vi "gyro -- async fitter.vi"(11 "fitter event pair":T9) -> ()   [LabVIEW 2021]
uses:
  lorentzian.ctl
  circle corners.ctl
  peak -- parameters -- complex fit.ctl
  wavepacket.ctl
  filter method control.ctl
  show-win- control.ctl
  server talk-to-back pair.ctl
  server talkback message type.ctl
  server talkto message type.ctl
  cursor winow.ctl
  plot refs -- filter related.ctl
  cursor window action.ctl
  publisher action.ctl
  arr action.ctl
  cursor action.ctl
  2Dwindow.ctl
  four-corner circle transformation.ctl
  filter - complex - four.vi
  linear interp iiii- complex - z-omega.vi
  peak -- PM find lorenzian - V3.vi
  Q -- check range -- i -- real.vi
  replace cursor action stack.vi
  Q -- range multiplier -- real -- V2.vi
  Q - not nan and gtr than zero - Real.vi
  Q - not nan -- real.vi
  array - smart min max.vi
  tale of three indices.vi
  filter -- window span logic.vi
  linear interp iiii- complex - z-omega - divide.vi
  linear interpolation iiii- complex.vi
  containing bix.vi
  <vilib>/Analysis/baseanly.llb/A x B.vi
  <vilib>/Analysis/baseanly.llb/Complex A x B.vi
  line -- complex.vi
  Q -- check range -- i -- integer.vi
  peak -- guess at omega -- dzdomega V2.vi
  command stack.vi
  tale of three indices -- check state.vi
  Q - not nan -- integer.vi
  peak -- z center from mult phase points.vi
  peak -- estimate for lorentzian.vi
  peak -- fake phase around center.vi
  peak -- get weights.vi
  peak -- four corner circle transformation logic.vi
  peak - fit phase around center - V2.vi
  array - generate range.vi
  circle center from three points.vi
  <vilib>/Utility/error.llb/Clear Errors.vi
  peak -- fit function -- minus arctan.vi
  <vilib>/Analysis/Matrix/Numeric/Conversions/Array To Matrix.vi
  <vilib>/Analysis/Matrix/Numeric/Conversions/Array To Matrix - RA2.vi
  <vilib>/Analysis/baseanly.llb/Inverse Matrix.vi
  <vilib>/Analysis/baseanly.llb/Real Inverse Matrix.vi
  <vilib>/gmath/NumericalOptimization/Nonlinear Curve Fit.vi
  <vilib>/gmath/NumericalOptimization/Nonlinear Curve Fit LM.vi
  KM_filter pipe - plot staff - more - V3.vi
panel:
  in  "Tab :  Fit controls":T1(tab)
  out "lorentzian":T2={"A (VHz)"=0.00528140496001674, "ω (Hz)"=0.00023844547824536982, "Γ (Hz)"=0.8041391285680035, "φ (rad)"=1.5732633738560469, "Q"=0.0002965226660092878, "Norm  Ampl"=nan, "z∞ (V)"=0.027690666556369502-1.7738793870681028e-05i, "4corners"={"z (-pi/2)"=0.03424221869371515+0.006566219331209036i, "z(inf)"=0.027690666556369502-1.7738793870681028e-05i, "z (pi/2)"=0.03427462468144921-0.0065692909312163265i, "z center"=0.03425842168758218-1.535800003645652e-06i, "z(0)"=0.040826176818794864+1.4667193863389723e-05i, "radius"=0.006567775117997019}} {"z∞ (V)" format="%#_4p"; "Q" format="%#_4p"; "φ (rad)" format="%#_3p"; "Γ (Hz)" format="%#_5p"; "ω (Hz)" format="%#_9p"; "A (VHz)" format="%#_3p"}
  in  "Plot: fragment - filter":cluster{dbl[], dbl[]}[](graph)=[{array[1567 elements], array[1567 elements]}, {array[1567 elements], array[1567 elements]}, {array[1567 elements], array[1567 elements]}, {array[1567 elements], array[1567 elements]}]
  out "Plot: phase around center":cluster{dbl[], dbl[]}[](graph)
  out "Plot: fragment":cluster{dbl[], dbl[]}[](graph)
  out "Plot: complex plane":cluster{dbl[], dbl[]}[](graph)=[{array[1567 elements], array[1567 elements]}, {[0.0408261968055792, 0.04077440793707446, 0.04061985807295371, 0.04036498455689775, 0.040013806896508845, 0.039571863373274695, 0.03904612370056097, 0.038444879107068015, 0.03777761157920133, 0.03705484432448167, 0.03628797581427619, 0.035489100023095875, 0.03467081569939291, 0.03384602767577145, 0.03302774335206849, 0.03222886756088818, 0.0314619990506827, 0.030739231795963037, 0.03007196426809635, 0.029470719674603397, 0.02894498000188967, 0.02850303647865552, 0.02815185881826662, 0.027896985302210662, 0.02774243543808991, 0.027690646569585163, 0.02774243543808991, 0.027896985302210662, 0.02815185881826662, 0.02850303647865552, 0.02894498000188967, 0.029470719674603397, 0.030071964268096354, 0.03073923179596304, 0.031461999050682705, 0.03222886756088818, 0.03302774335206849, 0.03384602767577145, 0.03467081569939291, 0.03548910002309588, 0.03628797581427619, 0.03705484432448167, 0.03777761157920133, 0.038444879107068015, 0.03904612370056097, 0.0395718633732747, 0.040013806896508845, 0.04036498455689775, 0.04061985807295371, 0.04077440793707446], [-1.535800003645652e-06, 0.0008216246928581006, 0.001631803453015174, 0.002416223477442565, 0.0031625139937652446, 0.0038589055547284595, 0.004494415649411666, 0.00505902190398638, 0.00554382014053853, 0.005941164801273261, 0.006244789523528591, 0.006449905964057936, 0.006553279314063525, 0.006553279314063525, 0.006449905964057935, 0.00624478952352859, 0.005941164801273261, 0.005543820140538529, 0.005059021903986379, 0.004494415649411665, 0.00385890555472846, 0.003162513993765244, 0.0024162234774425632, 0.001631803453015174, 0.0008216246928580996, -1.5358000036477643e-06, -0.0008246962928653923, -0.0016348750530224665, -0.0024192950774498587, -0.003165585593772537, -0.003861977154735753, -0.0044974872494189565, -0.005062093503993671, -0.005546891740545822, -0.005944236401280553, -0.006247861123535881, -0.006452977564065226, -0.006556350914070815, -0.006556350914070815, -0.0064529775640652254, -0.0062478611235358816, -0.005944236401280552, -0.00554689174054582, -0.005062093503993669, -0.004497487249418954, -0.0038619771547357476, -0.0031655855937725366, -0.0024192950774498557, -0.0016348750530224632, -0.0008246962928653888]}, {[0.027690666556369502, 0.02834744206949077, 0.029004217582612037, 0.029660993095733307, 0.030317768608854573, 0.030974544121975842, 0.03163131963509711, 0.03228809514821838, 0.032944870661339644, 0.03360164617446092, 0.03425842168758218, 0.03491519720070345, 0.035571972713824715, 0.03622874822694599, 0.036885523740067254, 0.03754229925318853, 0.03819907476630979, 0.03885585027943106, 0.039512625792552325, 0.0401694013056736], [-1.7738793870681028e-05, -1.611849448397749e-05, -1.4498195097273952e-05, -1.2877895710570416e-05, -1.1257596323866877e-05, -9.63729693716334e-06, -8.016997550459804e-06, -6.396698163756265e-06, -4.7763987770527285e-06, -3.1560993903491917e-06, -1.5358000036456533e-06, 8.449938305788346e-08, 1.7047987697614202e-06, 3.325098156464957e-06, 4.945397543168497e-06, 6.565696929872034e-06, 8.18599631657557e-06, 9.806295703279107e-06, 1.1426595089982644e-05, 1.304689447668618e-05]}, {[0.03424221869371515, 0.034243838993101856, 0.03424545929248856, 0.034247079591875264, 0.03424869989126197, 0.034250320190648664, 0.03425194049003537, 0.03425356078942207, 0.034255181088808775, 0.03425680138819548, 0.03425842168758218, 0.03426004198696889, 0.03426166228635559, 0.034263282585742294, 0.034264902885129, 0.0342665231845157, 0.0342681434839024, 0.0342697637832891, 0.034271384082675806, 0.03427300438206251], [0.006566219331209036, 0.005909443818087768, 0.005252668304966499, 0.004595892791845232, 0.003939117278723963, 0.003282341765602695, 0.0026255662524814274, 0.001968790739360159, 0.001312015226238891, 0.0006552397131176233, -1.5358000036453517e-06, -0.0006583113131249131, -0.0013150868262461809, -0.0019718623393674486, -0.002628637852488718, -0.003285413365609986, -0.003942188878731254, -0.0045989643918525214, -0.005255739904973789, -0.005912515418095059]}, {[0.161429891576008, 0.16228628660951472, 0.1630599306451906, 0.16375034018069645, 0.16435708373254648, 0.16487978210577106, 0.16531810863090154, 0.16567178936812785, 0.16594060327850202, 0.16612438236208033, 0.16622301176291782, 0.1662364298408495, 0.16616462821001343, 0.16600765174409163, 0.1657655985482655, 0.1654386198979033, 0.16502692014401782, 0.16453075658555388, 0.16395043930858472, 0.16328633099251824], [-0.035709224864324776, -0.0324095456256249, -0.02908948983727056, -0.02575113242605699, -0.022396559756697982, -0.019027868327915826, -0.015647163462197872, -0.012256557990038502, -0.008858170929488846, -0.005454126161839468, -0.0020465511042637103, 0.0013624246197488027, 0.004770670511337509, 0.008176056527763353, 0.011576454413616181, 0.01496973903090505, 0.01835378968720035, 0.021726491460997498, 0.02508573652347404, 0.028429425455814096]}, {[0.17590062231507544, 0.17685122080226792, 0.17770996568186812, 0.17847632026627963, 0.17914980560883315, 0.17973000080311247, 0.1802165432460073, 0.18060912886432848, 0.1809075123048438, 0.18111150708761575, 0.18122098572254536, 0.1812358797890495, 0.18115617997882147, 0.18098193610164828, 0.1807132570542813, 0.18035031075237923, 0.17989332402556635, 0.1793425824756714, 0.1786984302982356, 0.1779612700674018], [-0.039658649110643325, -0.03599600515568646, -0.03231074323061314, -0.02860516650416608, -0.024881590841177584, -0.021142343355229392, -0.017389760954282463, -0.01362618888018556, -0.00985397924297544, -0.006075489550884631, -0.00229308123697554, 0.0014908818166783503, 0.005274034756341815, 0.009054013234574502, 0.01282845488787114, 0.016595000813061783, 0.02035129704154957, 0.024094996010464404, 0.027823758029813368, 0.031535252744710834]}, {array[1567 elements], array[1567 elements]}]
  in  "scale gauge: Plot: complex plane":dbl(slide)=0.00275 min=0.0 max=0.3 step=1e-06 scale=1e-06..5000000000.0 scale format="%#_3p"
  out "Plot: phase":cluster{"omega out":dbl[], dbl[]}(graph)
  out "Plot: win omega":T4(graph)
  out "Plot: dz/domega":cluster{"omega out":dbl[], dbl[]}(graph)
  in  "Plot: complex plane - filter":cluster{dbl[], dbl[]}[](graph)=[{array[1567 elements], array[1567 elements]}, {array[1567 elements], array[1567 elements]}, {[0.041161284502408316, 0.04114804194794312, 0.04110836654686009, 0.041042414879841324, 0.04095044722798609, 0.040832826545600234, 0.04069001702778137, 0.04052258227845285, 0.040331183086076625, 0.04011657481582302, 0.03987960442848954, 0.03962120713793352, 0.039342402720210286, 0.039044291488982974, 0.038728049953087165, 0.038394926173388036, 0.03804623483725427, 0.037683352070087675, 0.03730771000438489, 0.0369207911277647, 0.03652412243226672, 0.03611926938801138, 0.0357078297650046, 0.0352914273274695, 0.03487170542559085, 0.034450320509962676, 0.0340289355943345, 0.03360921369245585, 0.03319281125492075, 0.03278137163191397, 0.03237651858765863, 0.03197984989216064, 0.03159293101554046, 0.031217288949837673, 0.030854406182671077, 0.030505714846537316, 0.030172591066838183, 0.029856349530942378, 0.029558238299715062, 0.02927943388199183, 0.02902103659143581, 0.02878406620410233, 0.028569457933848727, 0.0283780587414725, 0.028210623992143982, 0.028067814474325114, 0.027950193791939262, 0.027858226140084028, 0.02779227447306526, 0.027752599071982225, 0.02773935651751704, 0.027752599071982225, 0.02779227447306526, 0.027858226140084028, 0.027950193791939262, 0.028067814474325114, 0.028210623992143982, 0.0283780587414725, 0.028569457933848727, 0.028784066204102333, 0.02902103659143581, 0.029279433881991834, 0.029558238299715066, 0.029856349530942378, 0.030172591066838183, 0.030505714846537316, 0.03085440618267108, 0.031217288949837677, 0.03159293101554046, 0.03197984989216065, 0.03237651858765862, 0.03278137163191397, 0.03319281125492075, 0.033609213692455855, 0.0340289355943345, 0.034450320509962676, 0.03487170542559086, 0.0352914273274695, 0.035707829765004605, 0.03611926938801138, 0.03652412243226672, 0.03692079112776471, 0.03730771000438489, 0.03768335207008768, 0.03804623483725427, 0.03839492617338804, 0.03872804995308717, 0.039044291488982974, 0.03934240272021029, 0.03962120713793352, 0.03987960442848955, 0.04011657481582302, 0.040331183086076625, 0.04052258227845285, 0.04069001702778137, 0.04083282654560024, 0.04095044722798609, 0.041042414879841324, 0.04110836654686009, 0.04114804194794312], [0.0, 0.0004213849156281766, 0.0008411068175068247, 0.0012575092550419264, 0.0016689488780487088, 0.002073801922304048, 0.0024704706178020307, 0.002857389494422215, 0.0032330315601250014, 0.0035959143272915966, 0.003944605663425361, 0.004277729443124494, 0.004593970979020299, 0.004892082210247612, 0.005170886627970845, 0.005429283918526867, 0.005666254305860345, 0.005880862576113948, 0.006072261768490176, 0.006239696517818694, 0.006382506035637562, 0.0065001267180234135, 0.006592094369878648, 0.006658046036897418, 0.00669772143798045, 0.006710963992445636, 0.00669772143798045, 0.006658046036897418, 0.006592094369878648, 0.0065001267180234135, 0.006382506035637562, 0.006239696517818694, 0.006072261768490176, 0.005880862576113947, 0.005666254305860344, 0.005429283918526867, 0.005170886627970844, 0.004892082210247611, 0.004593970979020297, 0.004277729443124492, 0.003944605663425362, 0.0035959143272915966, 0.0032330315601250006, 0.002857389494422214, 0.002470470617802029, 0.0020738019223040458, 0.0016689488780487088, 0.001257509255041926, 0.0008411068175068236, 0.000421384915628175, -2.1584377821951928e-18, -0.0004213849156281764, -0.000841106817506825, -0.0012575092550419272, -0.00166894887804871, -0.00207380192230405, -0.002470470617802033, -0.0028573894944222147, -0.003233031560125002, -0.003595914327291598, -0.003944605663425363, -0.0042777294431244955, -0.004593970979020299, -0.004892082210247612, -0.005170886627970845, -0.005429283918526866, -0.0056662543058603465, -0.005880862576113948, -0.0060722617684901775, -0.006239696517818694, -0.006382506035637562, -0.006500126718023414, -0.006592094369878648, -0.006658046036897419, -0.006697721437980451, -0.006710963992445636, -0.00669772143798045, -0.006658046036897418, -0.006592094369878647, -0.0065001267180234135, -0.006382506035637563, -0.006239696517818693, -0.006072261768490176, -0.005880862576113946, -0.005666254305860345, -0.005429283918526863, -0.005170886627970843, -0.004892082210247612, -0.004593970979020296, -0.004277729443124492, -0.0039446056634253575, -0.003595914327291595, -0.0032330315601250014, -0.0028573894944222116, -0.00247047061780203, -0.0020738019223040436, -0.0016689488780487068, -0.0012575092550419268, -0.0008411068175068216, -0.00042138491562817583]}, {[-0.0011564988801927543, 0.004572526561840443, -0.002112059205125437], [0.00335441079091194, -0.0001946319203892838, 0.002611932143364084]}, {[-0.0013298665711747892, -0.00137040717662973, -0.0014109477820846707, -0.0014514883875396116, -0.0014920289929945525, -0.0015325695984494932, -0.001573110203904434, -0.001613650809359375, -0.0016541914148143159, -0.0016947320202692566, -0.0017352726257241974, -0.0017758132311791381, -0.001816353836634079, -0.00185689444208902, -0.0018974350475439608, -0.0019379756529989017, -0.001978516258453842, -0.002019056863908783, -0.002059597469363724, -0.002100138074818665], [0.002923118173286433, 0.002884411809776051, 0.002845705446265669, 0.0028069990827552867, 0.002768292719244905, 0.0027295863557345226, 0.0026908799922241403, 0.0026521736287137584, 0.002613467265203376, 0.0025747609016929943, 0.002536054538182612, 0.0024973481746722297, 0.002458641811161848, 0.0024199354476514656, 0.0023812290841410838, 0.0023425227206307015, 0.0023038163571203196, 0.0022651099936099373, 0.002226403630099555, 0.002187697266589173]}, {[0.004572526561840443, 0.004665772051033478, 0.0047590175402265145, 0.00485226302941955, 0.004945508518612586, 0.005038754007805622, 0.005131999496998658, 0.005225244986191694, 0.00531849047538473, 0.005411735964577766, 0.005504981453770801, 0.005598226942963838, 0.005691472432156874, 0.0057847179213499095, 0.005877963410542945, 0.0059712088997359814, 0.006064454388929017, 0.006157699878122053, 0.006250945367315089, 0.006344190856508124], [-0.0001946319203892838, -0.0001946319203892838, -0.0001946319203892838, -0.0001946319203892838, -0.0001946319203892838, -0.0001946319203892838, -0.0001946319203892838, -0.0001946319203892838, -0.0001946319203892838, -0.0001946319203892838, -0.0001946319203892838, -0.0001946319203892838, -0.0001946319203892838, -0.0001946319203892838, -0.0001946319203892838, -0.0001946319203892838, -0.0001946319203892838, -0.0001946319203892838, -0.0001946319203892838, -0.0001946319203892838]}]
  in  "parameters: complex fit":T5={"main VI path"=path "", "scale factor"=3.0, "# of grid points"=200, "parameters: wavepacket"={"R"=0.5, "wave number"=22.0, "delta k"=7.0, "radii vector"=[], "radial section"=[], "wave vector"=22.0, "wavepacket is"=TRUE}, "span"=0.27789, "interference ?"=enum."cp z center", "filter method"=enum."three"} {"span" min=0.0 max=0.5 step=1e-05 scale=0.0001..0.5 scale format="%#_5f"; "parameters: wavepacket"."delta k" format="%#_3f"; "parameters: wavepacket"."wave number" format="%#_3f"; "parameters: wavepacket"."R" format="%#_3f"}
  in  "win":T8={"cen (Hz)"=45005.0594236074, "win (Hz)"=127.23590686512762, "left (Hz)"=44941.44147017484, "right (Hz)"=45068.67737703997} {"right (Hz)" format="%#_3p"}
  out "circle frequency (Hz)":dbl=0.00023844547824536982 format="%#11_11f"
  out "circle gamma (Hz)":dbl=0.8041391285680035 format="%#11_11f"
  out "circle phase (rad)":dbl=1.5732633738560469 format="%#11_11f"
  out "circle Q":dbl=0.0002965226660092878 format="%#11_11f"
  in  "use fast fit!":bool
  in  "plot staff!":enum16{"plot", "do not plot", "a"}(ring)
  in  "cursor window":T10={"left"=0.0, "right "=0.0, "center"=0.0, "window"=0.0, "cursors"=[4, 5, 6], "relative"=0, "absolute"=0, "fixed vertical offset"=0.0, "vertical offset"=0.0, "skew"=0.0, "default window frac"=0.1, "kind"=enum."symmetric", "skew.left"=0.5, "skew.right"=0.5, "Plot ref"=refnum, "wing order"=enum."forw"}
  in  "tab":enum32{"complex plane"}(tab)
  out "# of points":dbl=953.475933538175
  out "center (kHz)":dbl=3399.029286744401
  out "win width (kHz)":dbl=76.27809365793496
  in  "ignore win":T8 {"right (Hz)" format="%#_3p"}
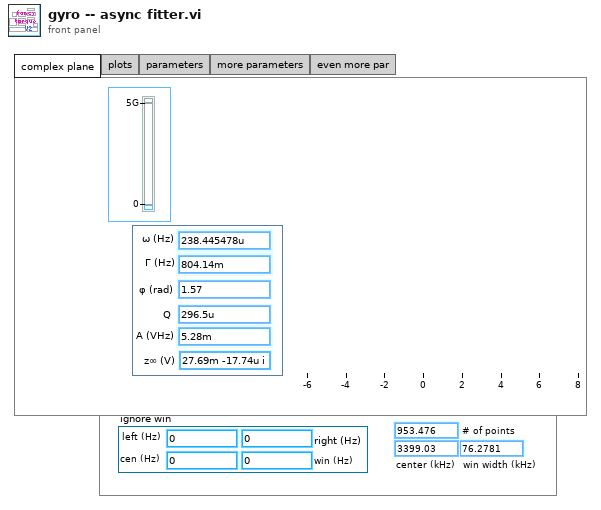
[diagram p1: front panel]
types:
  T1 = enum32{"complex plane", "plots", "parameters", "more parameters", "even more par"}
  T2 = typedef "lorentzian.ctl" = cluster{"A (VHz)":dbl, "ω (Hz)":dbl, "Γ (Hz)":dbl, "φ (rad)":dbl, "Q":dbl, "Norm  Ampl":dbl, "z∞ (V)":cdb, "4corners":T3}
  T3 = typedef "circle corners.ctl" = cluster{"z (-pi/2)":cdb, "z(inf)":cdb, "z (pi/2)":cdb, "z center":cdb, "z(0)":cdb, "radius":dbl}
  T4 = cluster{"omega out":dbl[], "win omega out":dbl[]}
  T5 = typedef "peak -- parameters -- complex fit.ctl" = cluster{"main VI path":path, "scale factor":dbl, "# of grid points":i32, "parameters: wavepacket":T6, "span":dbl, "interference ?":enum16{"cp z center", "pm zcenter", "fancy"}, "filter method":T7}
  T6 = typedef "wavepacket.ctl" = cluster{"R":dbl, "wave number":dbl, "delta k":dbl, "radii vector":dbl[], "radial section":cdb[], "wave vector":dbl, "wavepacket is":bool}
  T7 = typedef "filter method control.ctl" = enum16{"four", "five", "one", "two", "three", "zero", "minus one", "minus two"}
  T8 = typedef "show-win- control.ctl" = cluster{"cen (Hz)":dbl, "win (Hz)":dbl, "left (Hz)":dbl, "right (Hz)":dbl}
  T9 = typedef "server talk-to-back pair.ctl" = cluster{"talkback event":refnum<user-event>, "talkto event":refnum<user-event>}
  T10 = typedef "cursor winow.ctl" = cluster{"left":dbl, "right ":dbl, "center":dbl, "window":dbl, "cursors":i32[], "relative":i32, "absolute":i32, "fixed vertical offset":dbl, "vertical offset":dbl, "skew":dbl, "default window frac":dbl, "kind":enum16{"symmetric", "skewed", "fancy"}, "skew.left":dbl, "skew.right":dbl, "Plot ref":refnum<vi>, "wing order":enum16{"forw", "back"}}
  T11 = typedef "cursor window action.ctl" = enum16{"balance", "h. offset change", "cursor moves", "change center", "change window", "init", "check", "reset", "set y to middle", "idle", "-write all Y", "-write left.X", "-write center.X", "-write right.X", "-write all X", "-change center", "-change window", "-change skew", "-read cursor 2", "-read cursor 1", "-read cursor 0", "-read all cursors", "-reset", "-read plot scale", "-set y to middle", "-Q: center.Y is visible", "-Q: window is visible", "-parse center.Y", "-right left from center", "-left move", "-right move", "-set center.Y", "-empty", "-set cursors to default", "-check", "-write center.Y", "-copy cursor 1", "-copy cursor 0", "-copy cursor 2", "move right", "move left", "shrink", "broaden", "skew up", "skew down", "-write plot scale", "zoom X", "change cen&win", "zoom to all data", "color--red", "color--green", "color--yellow", "read", "zoom out", "zoom in", "slide right", "slide left", "set range aspect ratio to 1", "move to window range", "--move to window range"}
  T12 = enum16{"stop", "start", "update pars", "update request", "new", "launch", "exit", "get", "reset", "pause", "unpause"}
  T13 = typedef "plot refs -- filter related.ctl" = cluster{"Plot: complex plane - filter":refnum<vi>, "Plot: dz/domega":refnum<vi>, "Plot: fragment filter":refnum<vi>, "Plot: win omega":refnum<vi>, "Plot: phase":refnum<vi>, "Plot: phase around center":refnum<vi>, "Plot: complex plane":refnum<vi>, "Plot: fragment":refnum<vi>}
  T14 = typedef "arr action.ctl" = enum16{"select", "remove", "init", "check"}
  T15 = typedef "publisher action.ctl" = enum16{"set", "get", "init", "check"}
  T16 = typedef "server talkback message type.ctl" = cluster{"message":enum16{"new", "void"}}
  T17 = typedef "four-corner circle transformation.ctl" = enum16{"z(c) z(inf)", "z(c) z(zero)", "fix phase", "calculate lorentzian", "z(0) z(+-pi/2)", "shift to zcenter", "to  canonical", "get canonical phase", "get4corners", "update lorentzian -- from z0", "fake gamma normal", "fake gamma heat", "calculate complex slope", "get f0 given f and phi"}
  T18 = typedef "2Dwindow.ctl" = cluster{"window y":dbl, "center x":dbl, "center y":dbl, "window x":dbl}
  T19 = typedef "cursor action.ctl" = enum16{"range", "read", "write", "check", "zoom out", "smart zoom out", "zoom to aspect ratio 1", "zoom to win", "zoom out 20%", "zoom in 20%", "-empty", "smart zoom out&aspect", "move range left 20%", "move range right 20%", "move range up 20%", "move range down 20%", "zoom to X win", "zoom to Y win", "zoom out X", "zoom out Y", "zoom in X", "zoom in Y", "check plot scale", "set plot color", "set Xlabel", "set Ylabel", "set cursor color", "setlength", "empty", "hide plot", "unhide plot", "checklngth", "extend +1 if short", "extend +n if short"}
  T20 = typedef "eventvkey.ctl" = enum16{"ASCII", "Enter", "Return", "Shift", "Ctrl", "Alt", "Cmd", "Opt", "Caps", "NumLock", "Clear", "Break", "Up", "Down", "Left", "Right", "Insert", "Delete", "Home", "End", "PageUp", "PageDown", "Escape", "Help", "Pause", "ScrollLock", "F1", "F2", "F3", "F4", "F5", "F6", "F7", "F8", "F9", "F10", "F11", "F12", "F13", "F14", "F15", "F16", "F17", "F18", "F19", "F20", "F21", "F22", "F23", "F24", "Play", "VolumeUp", "VolumeDown", "Mute", "Two Byte Char"}
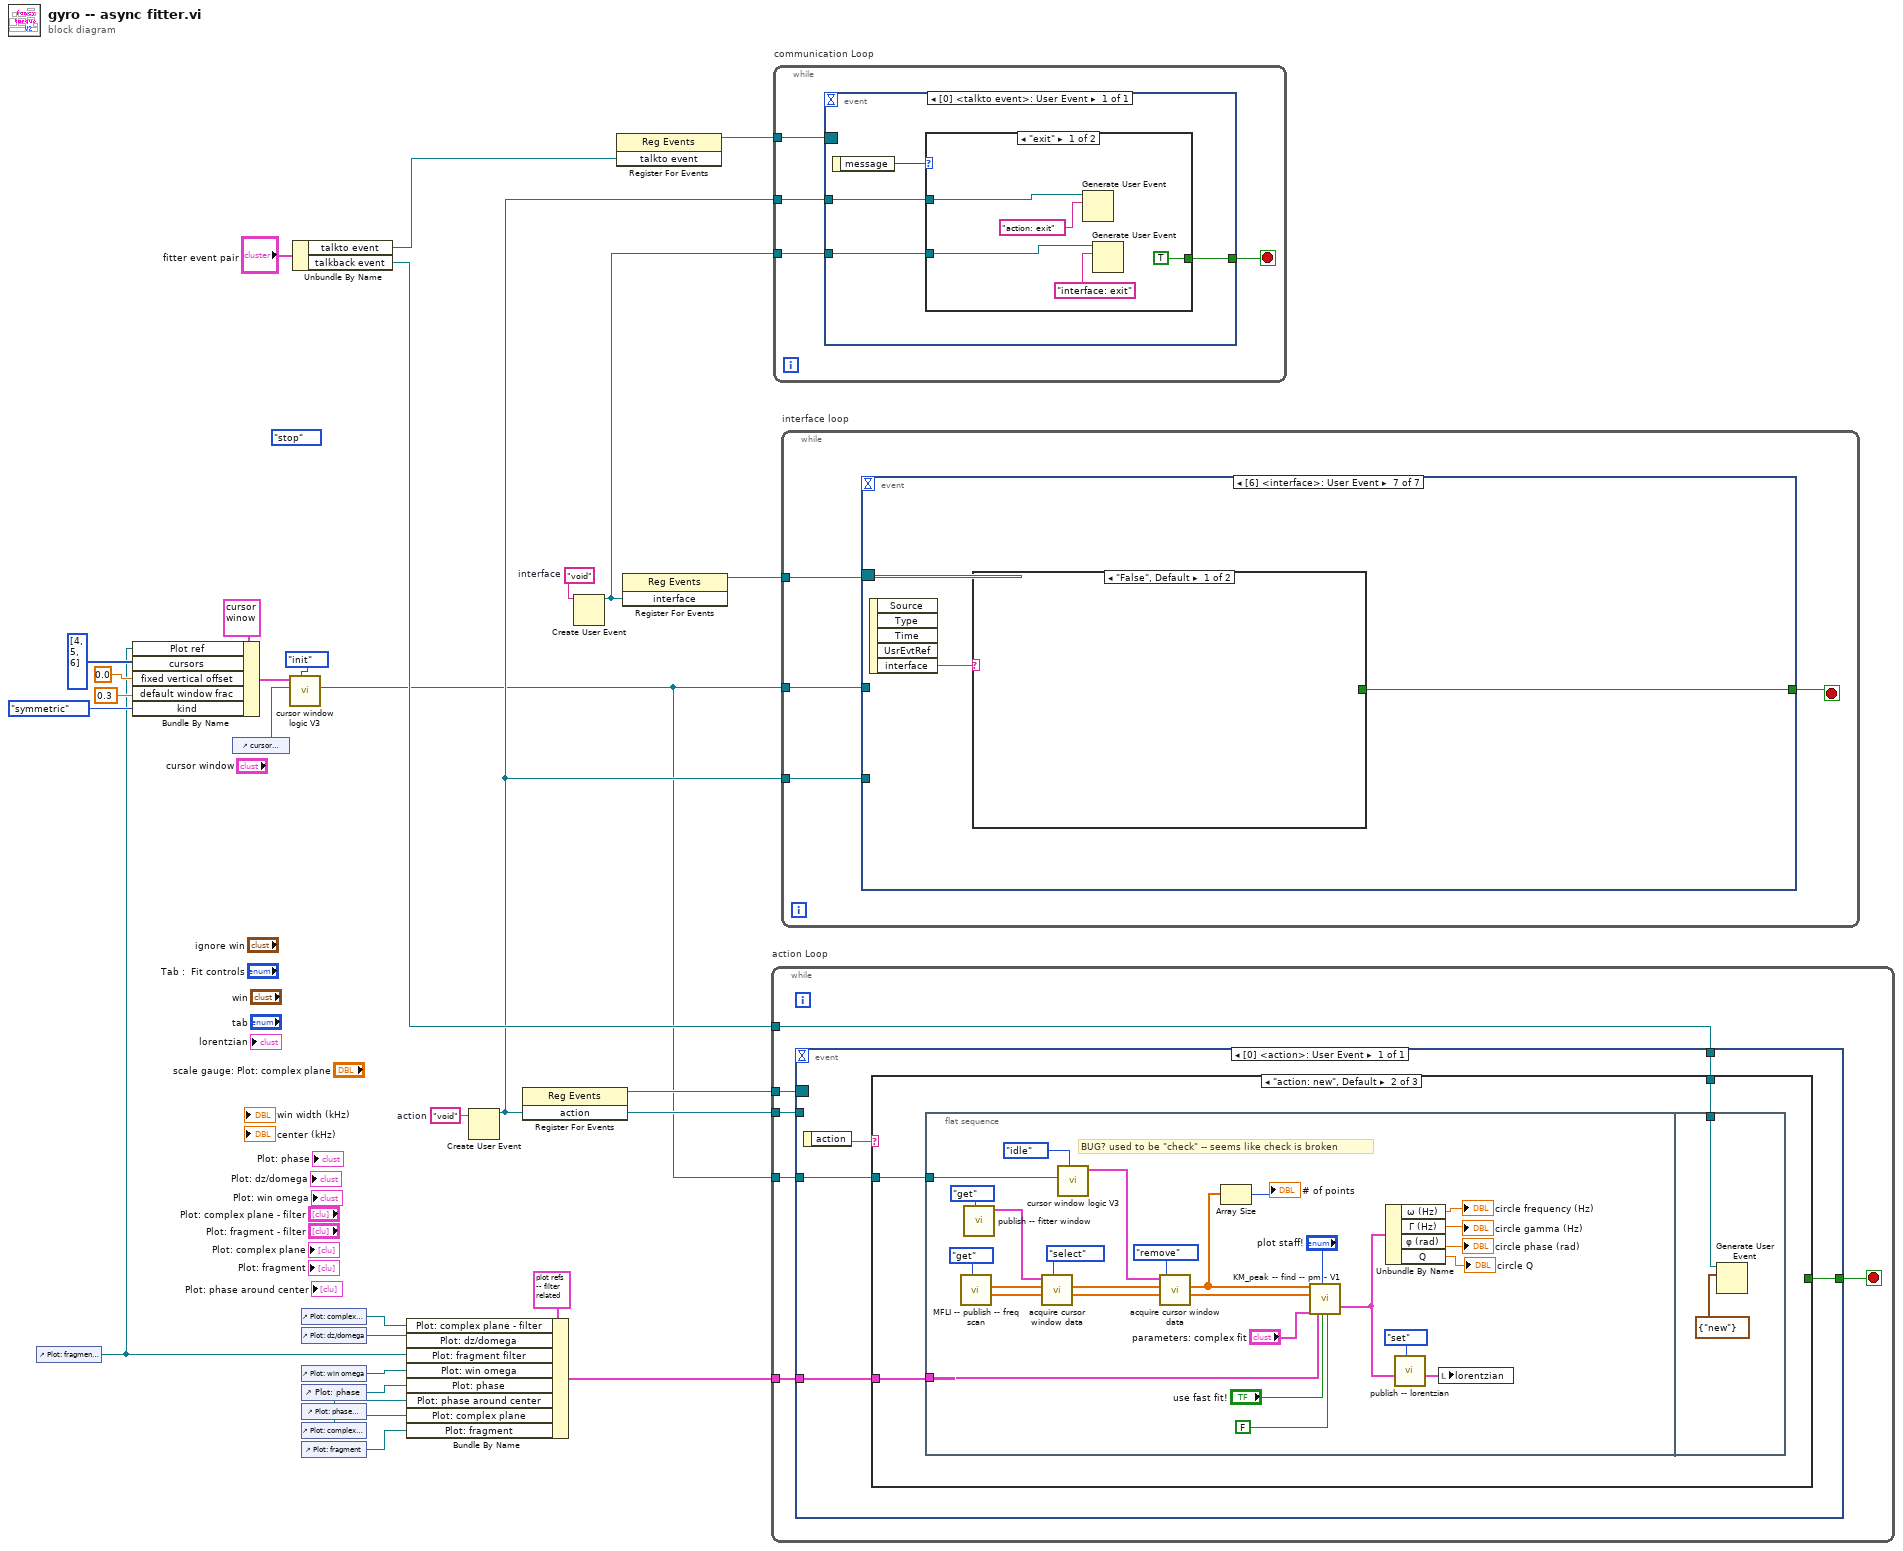
[diagram p0: block diagram]
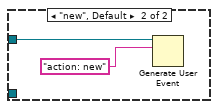
[diagram p2: hidden frame]
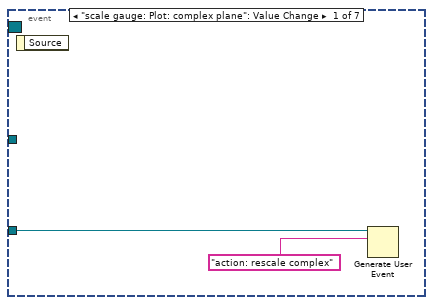
[diagram p3: hidden frame]
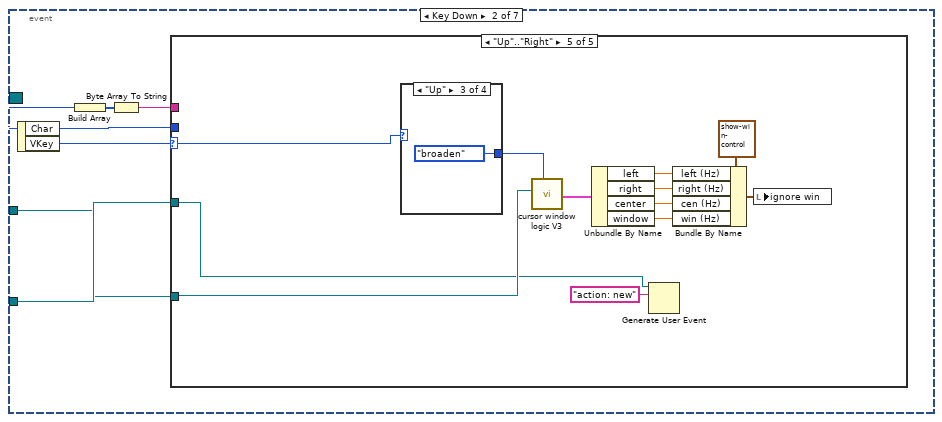
[diagram p4: hidden frame]
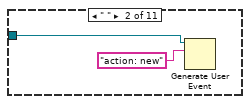
[diagram p6: hidden frame]
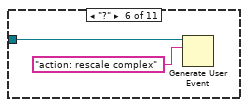
[diagram p10: hidden frame]
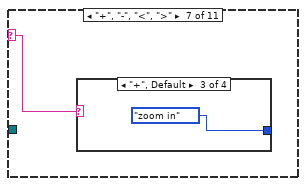
[diagram p11: hidden frame]
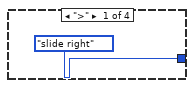
[diagram p12: hidden frame]
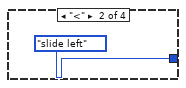
[diagram p13: hidden frame]
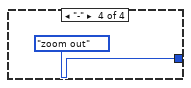
[diagram p14: hidden frame]
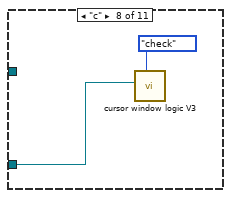
[diagram p15: hidden frame]
diagram:
  (unwired) T12."stop" ("message")
  w26 = "void"  # interface
  w28 = "void"  # action
  n1 = control-ref of="Plot: fragment - filter"() -> (w2:refnum<vi>)
  n2 = Bundle By Name(cluster=T10 {"left"=0.0, "right "=0.0, "center"=0.0, "window"=0.0, "cursors"=[], "relative"=0, "absolute"=0, "fixed vertical offset"=0.0, "vertical offset"=0.0, "skew"=0.0, "default window frac"=0.0, "kind"=enum."symmetric", "skew.left"=0.0, "skew.right"=0.0, "Plot ref"=refnum, "wing order"=enum."forw"} ("cursor bracket: All, data window"), "Plot ref"=w2, "cursors"=i32[] [4, 5, 6], "fixed vertical offset"=0.0, "default window frac"=0.3 ("fixed vertical offset"), "kind"=enum16{"symmetric", "skewed", "fancy"}."symmetric") -> (w6:T10)
  n3 = control-ref of="cursor window"() -> (w3:refnum<vi>)
  n4 = call "cursor window logic V3.vi"("cursor window action"=cursor_window_action."init", "cursor window in"=w3, "cursor window init"=w6) -> ("cursor window out"=w1:refnum<vi>)  [unwired: 7 in, 1 out]
  n5 = Unbundle By Name("fitter event pair") -> ("talkto event"=w14:refnum<user-event>, "talkback event"=w13:refnum<user-event>)
  n6 = control-ref of="Plot: complex plane - filter"() -> (w24:refnum<vi>)
  n7 = control-ref of="Plot: dz/domega"() -> (w23:refnum<vi>)
  n8 = control-ref of="Plot: win omega"() -> (w22:refnum<vi>)
  n9 = control-ref of="Plot: phase"() -> (w21:refnum<vi>)
  n10 = control-ref of="Plot: phase around center"() -> (w19:refnum<vi>)
  n11 = control-ref of="Plot: complex plane"() -> (w18:refnum<vi>)
  n12 = control-ref of="Plot: fragment"() -> (w17:refnum<vi>)
  n13 = Bundle By Name(cluster=T13 {"Plot: complex plane - filter"=refnum, "Plot: dz/domega"=refnum, "Plot: fragment filter"=refnum, "Plot: win omega"=refnum, "Plot: phase"=refnum, "Plot: phase around center"=refnum, "Plot: complex plane"=refnum, "Plot: fragment"=refnum} ("plots: filter related"), "Plot: complex plane - filter"=w24, "Plot: dz/domega"=w23, "Plot: fragment filter"=w2, "Plot: win omega"=w22, "Plot: phase"=w21, "Plot: phase around center"=w19, "Plot: complex plane"=w18, "Plot: fragment"=w17) -> (w20:T13)
  n14 = Create User Event(user event datatype=w28) -> (user event=w11:refnum<user-event>)  [unwired: 1 in, 1 out]
  n15 = register-events(w11) -> (reference out=w29:refnum<event-registration>)  [unwired: 2 in, 1 out]
  n16 = Create User Event(user event datatype=w26) -> (user event=w12:refnum<user-event>)  [unwired: 1 in, 1 out]
  n17 = register-events(w14) -> (reference out=w16:refnum<event-registration>)  [unwired: 2 in, 1 out]
  n18 = register-events(w12) -> (reference out=w27:refnum<event-registration>)  [unwired: 2 in, 1 out]
  n19 = while "action Loop" {
    tunnel: w29 -> [w35]
    tunnel: w11 -> [w34]
    tunnel: w20 -> [w33]
    tunnel: w13 -> [w32]
    tunnel: w1 -> [w30]
    stop <- w31 stop-if-true
    n20 = event shown="[0] <action>: User Event" {
      selector: w35 -> [_]
      dyn-events: _ -> [_]
      timeout: _ -> [_]
      tunnel: w34 -> [_]
      tunnel: w33 -> [w40]
      tunnel: w32 -> [w39]
      tunnel: [w37] -> w31
      tunnel: w30 -> [w36]
      event User Event {
        n21 = event-data() -> ("action"=w38:string)  [unwired: 1 in]
        n22 = case shown="\"action: new\", Default" w38 {
          tunnel: w40 -> [_ w44 _]
          tunnel: w39 -> [_ w43 _]
          tunnel: [TRUE _ _] -> w37
          tunnel: w36 -> [_ w42 _]
          frame "action: exit" {
          }
          frame "action: new", Default {
            n23 = flat-sequence {
              tunnel: w44 -> [w70]
              tunnel: w42 -> [w47]
              tunnel: w43 -> [w72]
              frame #0 {
                # "BUG? used to be \"check\" -- seems like check is broken"
                n24 = call "MFLI -- publish -- freq scan.vi"("publisher action"=publisher_action."get") -> ("Voltage out (V)"=w57:cdb[], "Freq out (Hz)"=w58:dbl[])  [unwired: 9 in]
                n25 = call "publish -- fitter window.vi"("publisher action"=publisher_action."get") -> ("win OUT"=w55:T10)  [unwired: 10 in]
                n26 = call "acquire cursor window data.vi"("arr action"=arr_action."select", "z in"=w57, "omega in"=w58, "cursor window"=w55) -> ("z out"=w50:cdb[], "omega  out"=w52:dbl[])  [unwired: 3 in, 3 out]
                n27 = call "cursor window logic V3.vi"("cursor window action"=cursor_window_action."idle", "cursor window in"=w47) -> ("cursor window out"=w48:T10)  [unwired: 8 in, 1 out]
                n28 = call "acquire cursor window data.vi"("arr action"=arr_action."remove", "z in"=w50, "omega in"=w52, "cursor window"=w48) -> ("z out"=w51:cdb[], "omega  out"=w46:dbl[])  [unwired: 3 in, 3 out]
                n29 = Array Size(array=w46) -> (size(s)=→"# of points":i32)
                n30 = call "KM_peak -- find -- pm - V1.vi"("omega in"=w46, "z in"=w51, "parameters: complex fit"="parameters: complex fit", "plots: filter related"=w70, "plot staff ?"="plot staff!", "just guess?"="use fast fit!", "subtract linear BG"=FALSE) -> ("pm lorentzian"=w60:T2)  [unwired: 10 in, 2 out]
                n31 = Unbundle By Name(w60) -> ("ω (Hz)"=→"circle frequency (Hz)":dbl, "Γ (Hz)"=→"circle gamma (Hz)":dbl, "φ (rad)"=→"circle phase (rad)":dbl, "Q"=→"circle Q":dbl)
                n32 = call "publish -- lorentzian.vi"("publisher action"=publisher_action."set", "lorentzian IN"=w60) -> ()  [unwired: 9 in, 1 out]
                n33 = local write "lorentzian"(w60) -> ()
              }
              frame #1 {
                n34 = Generate User Event(user event=w72, event data cluster=T16 {"message"=enum."new"} ("event data")) -> ()  [unwired: 2 in, 2 out]
              }
            }
          }
          frame "action: rescale complex" {
            n35 = local read "lorentzian"() -> (w82:T2)
            n36 = call "lorentzian transformations.vi"("4 corner circle transformation"=four-corner_circle_transformation."get4corners", "lorentzian in"=w82) -> ("lorentzian out"=w74:T2)  [unwired: 6 in, 3 out]
            n37 = local read "scale gauge: Plot: complex plane"() -> (w83:dbl)
            n38 = Unbundle By Name(w74) -> ("4corners.z center"=w77:cdb)
            n39 = control-ref of="Plot: complex plane"() -> (w78:refnum<vi>)
            n40 = Complex To Re/Im(x + iy=w77) -> (x=w79:dbl, y=w80:dbl)
            n41 = Bundle By Name(cluster=T18 {"window y"=0.0021014740628288917, "center x"=44850.89441339177, "center y"=2.5658109925320947, "window x"=17480.201988350764} ("window IN"), "window x"=w83, "window y"=w83, "center x"=w79, "center y"=w80) -> (w81:T18)
            n42 = call "replace cursor - plot ref - V2.vi"("Plot ref in"=w78, "window IN"=w81, "cursor action"=cursor_action."zoom to win") -> ()  [unwired: 13 in, 4 out]
          }
        }
      }
    }
  }
  n43 = while "communication Loop" {
    tunnel: w16 -> [w87]
    tunnel: w11 -> [w85]
    tunnel: w12 -> [w84]
    stop <- w86 stop-if-true
    n44 = event shown="[0] <talkto event>: User Event" {
      selector: w87 -> [_]
      dyn-events: _ -> [_]
      timeout: _ -> [_]
      tunnel: [w90] -> w86
      tunnel: w85 -> [w89]
      tunnel: w84 -> [w88]
      event User Event {
        n45 = event-data() -> ("message"=w91:T12)  [unwired: 1 in]
        n46 = case shown="\"exit\"" w91 {
          tunnel: [TRUE _] -> w90
          tunnel: w89 -> [w95 w98]
          tunnel: w88 -> [w92 _]
          frame "exit" {
            n47 = Generate User Event(user event=w95, event data cluster="action: exit" ("event data")) -> ()  [unwired: 2 in, 2 out]
            n48 = Generate User Event(user event=w92, event data cluster="interface: exit" ("event data")) -> ()  [unwired: 2 in, 2 out]
          }
          frame "new", Default {
            n49 = Generate User Event(user event=w98, event data cluster="action: new" ("event data")) -> ()  [unwired: 2 in, 2 out]
          }
        }
      }
    }
  }
  n50 = while "interface loop" {
    tunnel: w27 -> [w102]
    tunnel: w11 -> [w100]
    tunnel: w1 -> [w99]
    stop <- w101 stop-if-true
    n51 = event shown="[6] <interface>: User Event" {
      selector: w102 -> [_ _ _ _ _ _ _]
      dyn-events: _ -> [_ _ _ _ _ _ _]
      timeout: _ -> [_ _ _ _ _ _ _]
      tunnel: [_ _ _ _ _ _ w174] -> w101
      tunnel: w100 -> [w104 w106 w142 w157 w162 _ _]
      tunnel: w99 -> [_ w105 w141 _ w163 _ _]
      event "scale gauge: Plot: complex plane": Value Change {
        n52 = event-data() -> ()  [unwired: 1 in, 1 out]
        n53 = Generate User Event(user event=w104, event data cluster="action: rescale complex" ("event data")) -> ()  [unwired: 2 in, 2 out]
      }
      event Key Down {
        n54 = event-data() -> ("Char"=w108:i16, "VKey"=w110:T20)  [unwired: 1 in]
        n55 = Build Array(w108) -> (w109:i16[])
        n56 = Byte Array To String(unsigned byte array=w109) -> (string=w107:string)
        n57 = case shown="\"Up\"..\"Right\"" w110 {
          selector: w110 -> [_ _ _ _ w128]
          tunnel: w108 -> [_ _ _ _ _]
          tunnel: w107 -> [w113 _ _ _ _]
          tunnel: w106 -> [w112 _ _ _ w126]
          tunnel: w105 -> [w111 _ _ _ w127]
          frame "ASCII", Default {
            n58 = case shown="\"0\", Default" w113 {
              selector: w113 -> [_ _ _ _ _ _ w118 _ _ _ _]
              tunnel: w112 -> [_ w114 _ _ _ w116 _ _ _ _ _]
              tunnel: w111 -> [_ _ _ _ _ _ _ w123 _ _ _]
              frame "0", Default {
              }
              frame " " {
                n59 = Generate User Event(user event=w114, event data cluster="action: new" ("event data")) -> ()  [unwired: 2 in, 2 out]
              }
              frame "s" {
              }
              frame "l" {
              }
              frame "p" {
              }
              frame "?" {
                n60 = Generate User Event(user event=w116, event data cluster="action: rescale complex" ("event data")) -> ()  [unwired: 2 in, 2 out]
              }
              frame "+", "-", "<", ">" {
                n61 = case shown="\"+\", Default" w118 {
                  tunnel: [cursor_window_action."slide right" ("cursor window action") cursor_window_action."slide left" ("cursor window action") cursor_window_action."zoom in" ("cursor window action") cursor_window_action."zoom out" ("cursor window action")] -> _
                  frame ">" {
                  }
                  frame "<" {
                  }
                  frame "+", Default {
                  }
                  frame "-" {
                  }
                }
              }
              frame "c" {
                n62 = call "cursor window logic V3.vi"("cursor window action"=cursor_window_action."check", "cursor window in"=w123) -> ()  [unwired: 8 in, 2 out]
              }
              frame "t" {
              }
              frame "r" {
              }
              frame "d" {
              }
            }
          }
          frame "Escape" {
          }
          frame "PageUp" {
          }
          frame "PageDown" {
          }
          frame "Up".."Right" {
            n63 = case shown="\"Up\"" w128 {
              tunnel: [cursor_window_action."move right" ("cursor window action") cursor_window_action."move left" ("cursor window action") cursor_window_action."broaden" ("cursor window action") cursor_window_action."shrink" ("cursor window action")] -> w136
              frame "Right", Default {
              }
              frame "Left" {
              }
              frame "Up" {
              }
              frame "Down" {
              }
            }
            n64 = call "cursor window logic V3.vi"("cursor window action"=w136, "cursor window in"=w127) -> ("cursor window out"=w135:T10)  [unwired: 8 in, 1 out]
            n65 = Unbundle By Name(w135) -> ("left"=w132:dbl, "right"=w131:dbl, "center"=w130:dbl, "window"=w129:dbl)
            n66 = Generate User Event(user event=w126, event data cluster="action: new" ("event data")) -> ()  [unwired: 2 in, 2 out]
            n67 = Bundle By Name(cluster=T8 {"cen (Hz)"=-0.35260838541595674, "win (Hz)"=17.234446484426172, "left (Hz)"=-8.969831627629043, "right (Hz)"=8.26461485679713} ("win"), "left (Hz)"=w132, "right (Hz)"=w131, "cen (Hz)"=w130, "win (Hz)"=w129) -> (w134:T8)
            n68 = local write "ignore win"(w134) -> ()
          }
        }
      }
      event "Plot: fragment - filter": Cursor Move {
        n69 = event-data() -> ("CursIdx"=w143:i32)  [unwired: 1 in]
        n70 = case shown="4..6" w143 {
          selector: w143 -> [w153 _]
          tunnel: w141 -> [w155 _]
          tunnel: w142 -> [w151 _]
          frame 4..6 {
            w150 = "action: new"  # event data
            n71 = call "cursor window logic V3.vi"("CursIdx"=w153, "cursor window action"=cursor_window_action."cursor moves", "cursor window in"=w155) -> ("cursor window out"=w152:T10)  [unwired: 7 in, 1 out]
            n72 = Unbundle By Name(w152) -> ("left"=w147:dbl, "right"=w146:dbl, "center"=w145:dbl, "window"=w144:dbl)
            n73 = Generate User Event(user event=w151, event data cluster=w150) -> ()  [unwired: 2 in, 2 out]
            n74 = Bundle By Name(cluster=T8 {"cen (Hz)"=-0.35260838541595674, "win (Hz)"=17.234446484426172, "left (Hz)"=-8.969831627629043, "right (Hz)"=8.26461485679713} ("win"), "left (Hz)"=w147, "right (Hz)"=w146, "cen (Hz)"=w145, "win (Hz)"=w144) -> (w148:T8)
            n75 = local write "ignore win"(w148) -> ()
          }
          frame 3, Default {
          }
        }
      }
      event "Plot: fragment - filter": Cursor Release {
        n76 = event-data() -> ("CursIdx"=w156:i32)  [unwired: 1 in]
        n77 = case shown="3, Default" w156 {
          tunnel: w157 -> [_ w158]
          frame 3, Default {
          }
          frame 4..6 {
            w159 = "action: fit"  # event data
            n78 = Generate User Event(user event=w158, event data cluster=w159) -> ()  [unwired: 2 in, 2 out]
          }
        }
      }
      event Value Change {
        n79 = event-data() -> ("NewVal"=w160:T8)  [unwired: 1 in]
        n80 = in-place {
          in-place-border: w163 -> [w170]
          n81 = in-place-cluster #1(w160) -> ("cen (Hz)"=w165:dbl, "win (Hz)"=w166:dbl)  [unwired: 2 out]
          n82 = call "cursor window logic V3.vi"("cursor window action"=cursor_window_action."change center", "center"=w165, "cursor window in"=w170) -> ("cursor window out"=w171:refnum<vi>)  [unwired: 7 in, 1 out]
          n83 = call "cursor window logic V3.vi"("cursor window action"=cursor_window_action."change window", "window"=w166, "cursor window in"=w171) -> ("cursor window out"=w169:T10)  [unwired: 7 in, 1 out]
          n84 = Unbundle By Name(w169) -> ("left"=w168:dbl, "right"=w167:dbl)
          n85 = in-place-cluster #1("left (Hz)"=w168, "right (Hz)"=w167, "cen (Hz)"=w165, "win (Hz)"=w166) -> (w164:T8)
        }
        n86 = Generate User Event(user event=w162, event data cluster="action: new" ("event data")) -> ()  [unwired: 2 in, 2 out]
        n87 = local write "ignore win"(w164) -> ()
      }
      event Timeout {
        n88 = event-data() -> ()  [unwired: 1 in, 3 out]
      }
      event User Event {
        n89 = event-data() -> ("interface"=w175:string)  [unwired: 1 in, 4 out]
        n90 = case shown="\"False\", Default" w175 {
          tunnel: [_ TRUE] -> w174
          frame "False", Default {
          }
          frame "interface: exit" {
          }
        }
      }
    }
  }
